vi "Q Learning (SubVI).vi"(4 "# action":i32, 5 "Mode":enum16{"Algorithm test", "Flappy Bird"}(ring), 6 "# state":i32, 7 "Q option":i32, 8 "alpha":dbl=1.0 format="%#_13g", 9 "Gamma":dbl format="%#_13g", 10 "Action":i32, 11 "State":i32) -> (1 "Next Action":i32, 3 "Q":dbl[][](array[numeric]))   [LabVIEW 2013]
doc: "Calculate the cumulative experience Q with Q-Learning. This vi works only for discrete states and actions."
panel:
  out "Best rewarded action":i32
  out "Reward":dbl format="%#_13g"
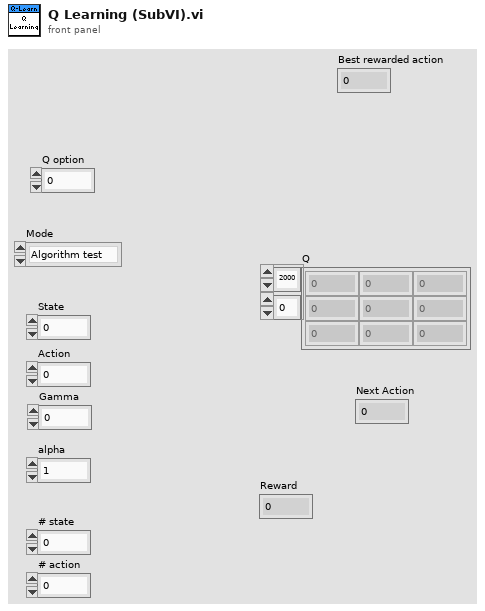
[diagram p1: front panel]
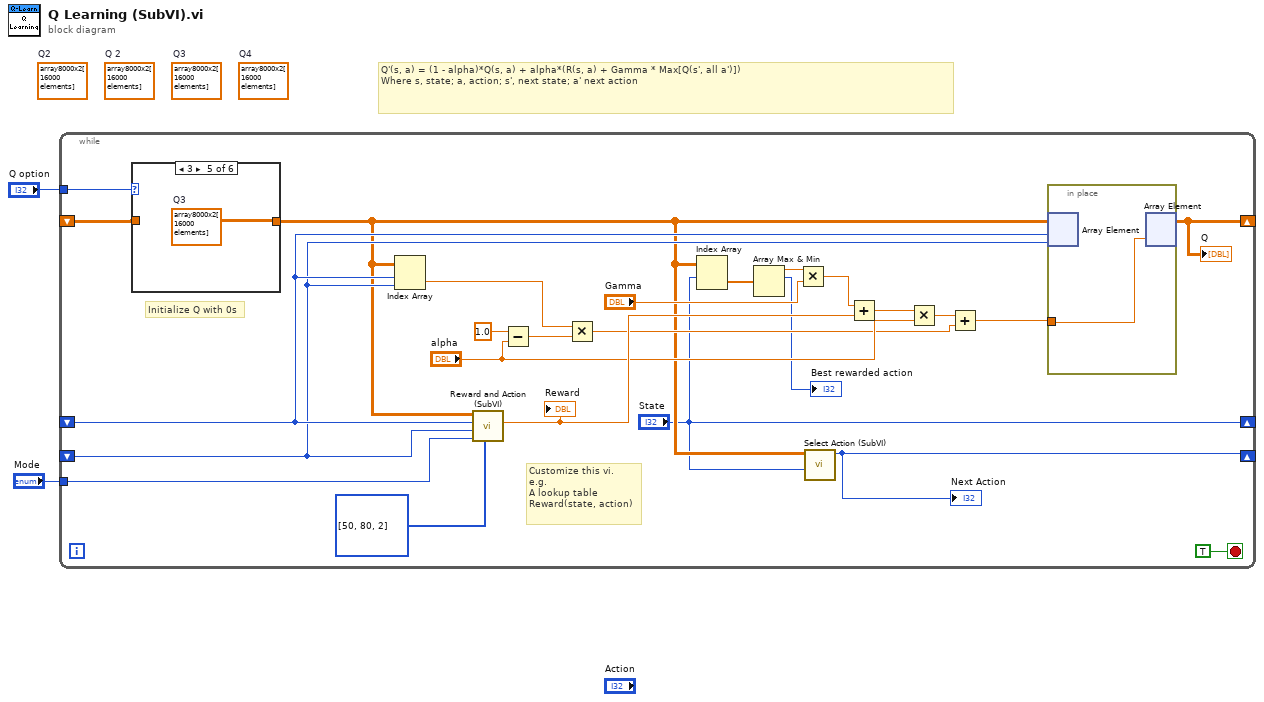
[diagram p0: block diagram]
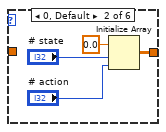
[diagram p3: hidden frame]
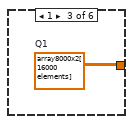
[diagram p4: hidden frame]
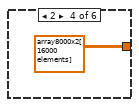
[diagram p5: hidden frame]
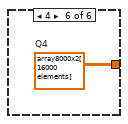
[diagram p6: hidden frame]
diagram:
  (unwired) dbl[][] array8000x2[16000 elements]  # Q3
  (unwired) dbl[][] array8000x2[16000 elements]  # Q2
  (unwired) dbl[][] array8000x2[16000 elements]  # Q4
  (unwired) dbl[][] array8000x2[16000 elements]  # Q 2
  # "Q'(s, a) = (1 - alpha)*Q(s, a) + alpha*(R(s, a) + Gamma * Max[Q(s', all a')])\nWhere s, state; a, action; s', next state; a' next action"
  n1 = while {
    shift-right: ["State"] -> _
    shift-left: _ -> [w11]
    shift-right: [w6] -> _
    shift-left: _ -> [w10]
    shift-right: [w22] -> _
    shift-left: _ -> [w20]
    tunnel: "Mode" -> [w8]
    tunnel: "Q option" -> [w3]
    stop <- TRUE stop-if-true
    # "Customize this vi.\ne.g. \nA lookup table\nReward(state, action)"
    # "Initialize Q with 0s"
    n2 = case shown="3" w3 {
      tunnel: [w28 w29 w33 dbl[][] array8000x2[16000 elements] ("Q") w35 w36] -> w7
      tunnel: w20 -> [w28 _ _ _ _ _]
      frame -1 {
      }
      frame 0, Default {
        n3 = Initialize Array(0.0 ("element"), "# state", "# action") -> (w29:dbl[][])
      }
      frame 1 {
        w33 = dbl[][] array8000x2[16000 elements]  # Q1
      }
      frame 2 {
      }
      frame 3 {
        w35 = dbl[][] array8000x2[16000 elements]  # Q3
      }
      frame 4 {
        w36 = dbl[][] array8000x2[16000 elements]  # Q4
      }
    }
    n4 = Index Array(array=w7, index (row)=w11, index (col)=w10) -> (element=w16:dbl)
    n5 = call "Reward and Action (SubVI).vi"("# each state"=i32[] [50, 80, 2], "Object"=w8, "Action"=w10, "State"=w11, "Q"=w7) -> ("Reward"=w24:dbl)  [unwired: 6 in]
    "Reward" <- w24
    n6 = Subtract(x=1.0, y="alpha") -> (x-y=w17:dbl)
    n7 = Multiply(x=w16, y=w17) -> (x*y=w12:dbl)
    n8 = Index Array(array=w7, index (row)="State") -> (element=w26:dbl[])  [unwired: 1 in]
    n9 = Array Max & Min(array=w26) -> (max value=w27:dbl, max index (indices)=→"Best rewarded action":i32)  [unwired: 2 out]
    n10 = Multiply(x=w27, y="Gamma") -> (x*y=w23:dbl)
    n11 = call "Select Action (SubVI).vi"("State"="State", "Q"=w7) -> ("Action"=w6:i32)  [unwired: 9 in]
    "Next Action" <- w6
    n12 = Add(x=w23, y=w24) -> (x+y=w21:dbl)
    n13 = Multiply(x=w21, y="alpha") -> (x*y=w15:dbl)
    n14 = Add(x=w15, y=w12) -> (x+y=w13:dbl)
    n15 = in-place {
      in-place-border: w13 -> [w37]
      n16 = in-place-array #1(w7, w11, w10) -> ()  [unwired: 1 out]
      n17 = in-place-array #1(w37) -> (w22:dbl[][])  [unwired: 2 out]
    }
    "Q" <- w22
  }
